vi "Identify_PID_Loops_Tags_Names_TT.vi"(8 "error in":errorcluster, 10 "PID_Loop Names":string, 11 "Tags":string[](array[string])=["MFC390LSP_CO", "MFC390HSP_CO", "MFC660LSP_H2", "MFC660HSP_H2", "HTR660SP", "HTR661SP", "HTR662SP", "MFC760LSP_N2", "MFC760HSP_N2", "MFC160LSP_O2", "MFC160HSP_O2", "MFC380LSP_CO2", "MFC380HSP_CO2", "MFC260LSP_CH4", "MFC260HSP_CH4", "CV760_N2", "CV460", "CV462", "CV461", "CV661", "CV160L_O2", "CV160H_O2", "CV760L_N2", "CV760H_N2", "CV380L_CO2", "CV380H_CO2", "CV260L_CH4", "CV260H_CH4", "CV390L_CO", "CV390H_CO", "CV660L_H2", "HTR660E", "HTR660RST", "HTR661E", "HTR661RST", "HTR662E", "HTR662RST", "PMP460", "PMP461", "DATE", "TIME", "ONLOAD_TIME", "H2UTIL", "O2UTIL", "CELL", "VT_AVG", "VT_MIN", "VT_MAX", "SD1_BP", "SD1_A", "SD1_B", "SD1_C", "SD1_D", "SDOUT", "AN_DR_SAT", "AN_SAT_MIN_FL", "AN_SAT_TOT_FL", "PCV662SP", "PMP440_SELECT", "PMP441_SELECT", "MFC760SP_N2", "MFC760LSP_N2_MAX", "CV760L", "CV760H", "MFC760_N2", "MFC760LSP_N2", "MFC760HSP_N2", "PID_001_SP", "PID_001_FB", "PID_001_OUT", "PID_001_UPD", "PID_001_OUTH", "PID_001_OUTL", "PID_001_AM", "PID_001_ERR", "PID_001_P", "PID_001_I", "PID_001_D", "PID_001_BUMP", "PID_001_SPMAX", "PID_001_SPMIN", "PID_002_SP", "PID_002_FB", "PID_002_OUT", "PID_002_UPD"]) -> (0 "error out":errorcluster, 2 "PID_Loop Names Out":string, 3 "PID Tag Set":string[](array[string]))   [LabVIEW 2010]
panel:
  in  "Search String (!PID)":string="!PID_"
  # "Find PID Parameters from Tag List by TekTHINK"
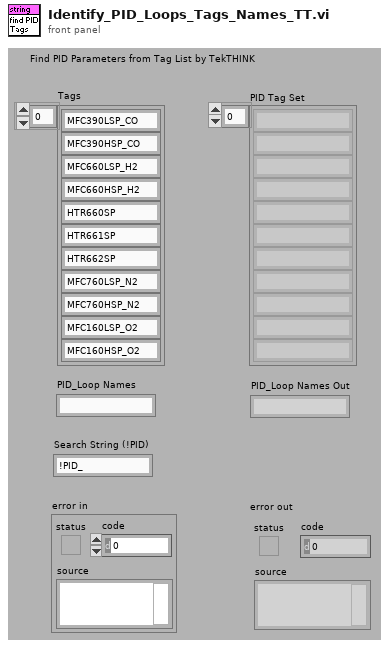
[diagram p1: front panel]
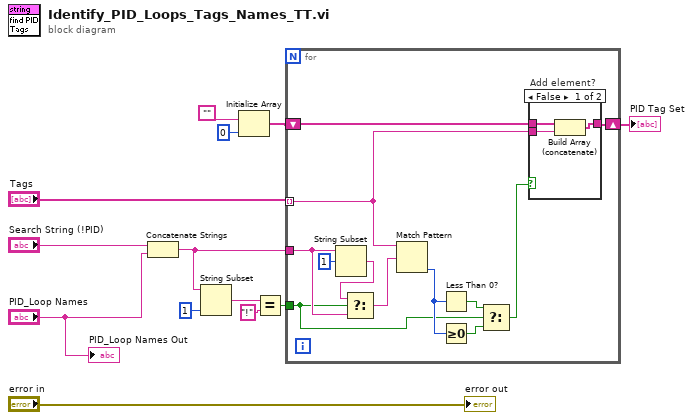
[diagram p0: block diagram]
diagram:
  n1 = Concatenate Strings("Search String (!PID)", "PID_Loop Names") -> (w4:string)
  n2 = String Subset(string=w4, length (rest)=1 ("length (rest)")) -> (substring=w9:string)  [unwired: 1 in]
  n3 = Initialize Array("", 0 ("dimension size")) -> (w11:string[])
  n4 = Equal?(x=w9, y="!") -> (x = y?=w7:bool)
  n5 = for {
    tunnel: w4 -> [w18]
    tunnel: "Tags" -> [w15] mode=indexing
    shift-right: [w24] -> w5
    shift-left: w11 -> [w25]
    tunnel: w7 -> [w16]
    n6 = String Subset(string=w18, offset (0)=1) -> (substring=w19:string)  [unwired: 1 in]
    n7 = Select(t=w19, s=w16, f=w18) -> (s? t:f=w14:string)
    n8 = Match Pattern(string=w15, regular expression=w14) -> (offset past match=w17:i32)  [unwired: 1 in, 3 out]
    n9 = Less Than 0?(x=w17) -> (x < 0?=w21:bool)
    n10 = Greater Or Equal To 0?(x=w17) -> (x >= 0?=w22:bool)
    n11 = Select(t=w21, s=w16, f=w22) -> (s? t:f=w23:bool)
    n12 = case "Add element?" shown="False" w23 {
      tunnel: w25 -> [w28 w29]
      tunnel: w15 -> [w26 _]
      tunnel: [w27 w29] -> w24
      frame False {
        n13 = Build Array (concatenate)(w28, w26) -> (w27:string[])
      }
      frame True {
      }
    }
  }
  "PID Tag Set" <- w5
  "error out" <- "error in"
  "PID_Loop Names Out" <- "PID_Loop Names"
